vi "niScope Digitizing Process.vi"(8 "error in":errorcluster, 11 "niScope session":variant) -> (0 "error out":errorcluster, 3 "auxiliary data out":variant)   [LabVIEW 2018, in "niScope Virtual Digitizer.lvlib"]
doc: "This is called assynchronously! It is process where niScope digitizers digitize samples, then fetching them and returning them via queue to the calling process. It handles both single shot and continuous sampling. For single shot sampling it returns the data in blocks of predifined size after all sampling is done. For streaming mode it streams the data blocks continuously. In any case the calling process must take the data from queue in parallel with this VI otherwise it will overflow! The function also returnes status in the data packet which may be used to determine progess of the digitizing and state of the memory buffer.\nThis VI also returns auxiliary data, i.e. structure with scaling factors, time stamps and measured temperature during sampling."
uses:
  niScope Virtual Digitizer.lvlib
  niScope Session.ctl
  niScope Virtual Channel Config.ctl
  niScope Virtual Channel Mode.ctl
  niScope Virtual Channel Input Z.ctl
  niScope Virtual Channel Coupling.ctl
  niScope Type.ctl
  niScope Digitizing Process Options.ctl
  niScope Data Packet.ctl
  niScope Trigger Setup.ctl
  <instrlib>/niScope/Controls/niScope trigger coupling.ctl
  <instrlib>/niScope/Controls/niScope trigger slope.ctl
  niScope Record Aux Data.ctl
  <vilib>/Analysis/baseanly.llb/Mean (DBL).vi
  <vilib>/Utility/error.llb/Error Cluster From Error Code.vi
  <instrlib>/niScope/Acquire/Fetch/niScope Fetch Binary 32.vi
  <instrlib>/niScope/Acquire/Fetch/niScope Fetch Binary 16.vi
  <vilib>/ErrorRing/Error Ring.xnode
  <vilib>/Analysis/NI_AALBase.lvlib
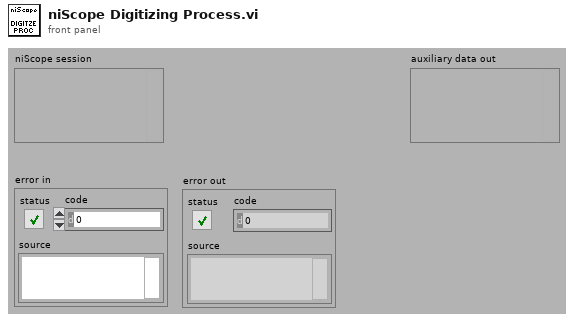
[diagram p1: front panel]
types:
  T1 = typedef "niScope Virtual Digitizer.lvlib/niScope Session.ctl" = cluster{"channel cfg":T2[], "sessions":refnum<k20>[], "multi cards":bool, "channels":i32, "type":T6, "memory [B/chn]":i32, "ext. clock [Hz]":dbl, "samples count":i64, "use streaming":bool, "proc setup":T7, "sample width [B]":i32, "ranges [V]":dbl[], "trigger setup":T8, "fs [Hz]":dbl, "bitres [bit]":i32}
  T2 = typedef "niScope Virtual Digitizer.lvlib/niScope Virtual Channel Config.ctl" = cluster{"Address":refnum<k15>, "Channel":i32, "Mode":T3, "Input Z":T4, "Coupling":T5, "Range [Vpk]":dbl, "btn clr":bool, "btn up":bool, "btn down":bool}
  T3 = typedef "niScope Virtual Digitizer.lvlib/niScope Virtual Channel Mode.ctl" = enum16{"Single ended", "Unbal. differential", "Differential"}
  T4 = typedef "niScope Virtual Digitizer.lvlib/niScope Virtual Channel Input Z.ctl" = enum16{"1 MOhm", "50 Ohm"}
  T5 = typedef "niScope Virtual Digitizer.lvlib/niScope Virtual Channel Coupling.ctl" = enum16{"AC", "DC", "GND"}
  T6 = typedef "niScope Virtual Digitizer.lvlib/niScope Type.ctl" = enum16{"n/a", "5922"}
  T7 = typedef "niScope Virtual Digitizer.lvlib/niScope Digitizing Process Options.ctl" = cluster{"packet size [smpl]":i64, "current timeout [s]":dbl, "blk2blk timeout [s]":dbl, "event time":timestamp, "temp sampl T [s]":dbl, "data queue":refnum<queue>, "stop notifier":refnum<notifier>, "proc ref":refnum<vi>}
  T8 = typedef "niScope Virtual Digitizer.lvlib/niScope Trigger Setup.ctl" = cluster{"coupling":T9, "level [V]":dbl, "slope":T10, "mode":enum16{"Immediate", "External", "Level"}}
  T9 = typedef "niScope trigger coupling.ctl" = u16
  T10 = typedef "niScope trigger slope.ctl" = i32
  T11 = typedef "niScope Virtual Digitizer.lvlib/niScope Data Packet.ctl" = cluster{"int32":i32[][], "card buffer [%]":dbl, "all done?":bool, "offset [smpl]":i64, "sampling?":bool, "queue buffer [%]":dbl, "int16":i16[][], "is int16?":bool, "count [smpl]":i32, "valid?":bool}
  T12 = typedef "niScope Virtual Digitizer.lvlib/niScope Record Aux Data.ctl" = cluster{"T smpl":i64[], "T [deg C]":dbl[][], "time stamp [s]":dbl[], "offset":dbl[], "gain":dbl[], "increment [s]":dbl, "valid?":bool, "abs timestamp":timestamp}
  T13 = cluster{"actualSamples":i32, "absoluteInitialX":dbl, "relativeInitialX":dbl, "xIncrement":dbl, "offset":dbl, "gain":dbl, "reserved1":dbl, "reserved2":dbl}
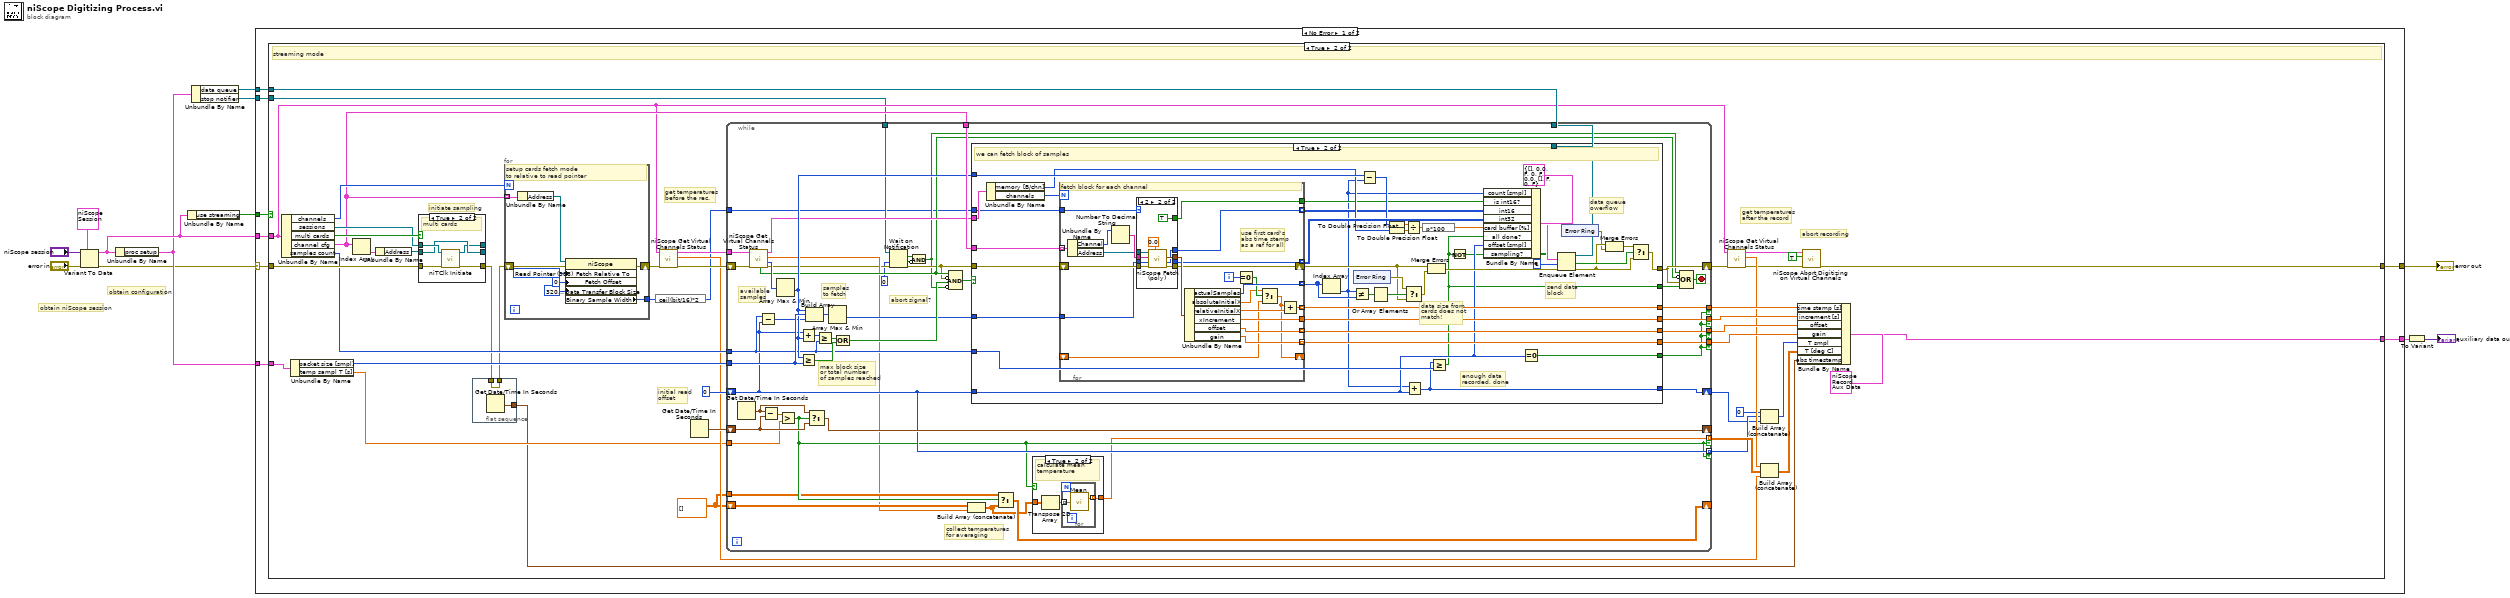
[diagram p0: block diagram]
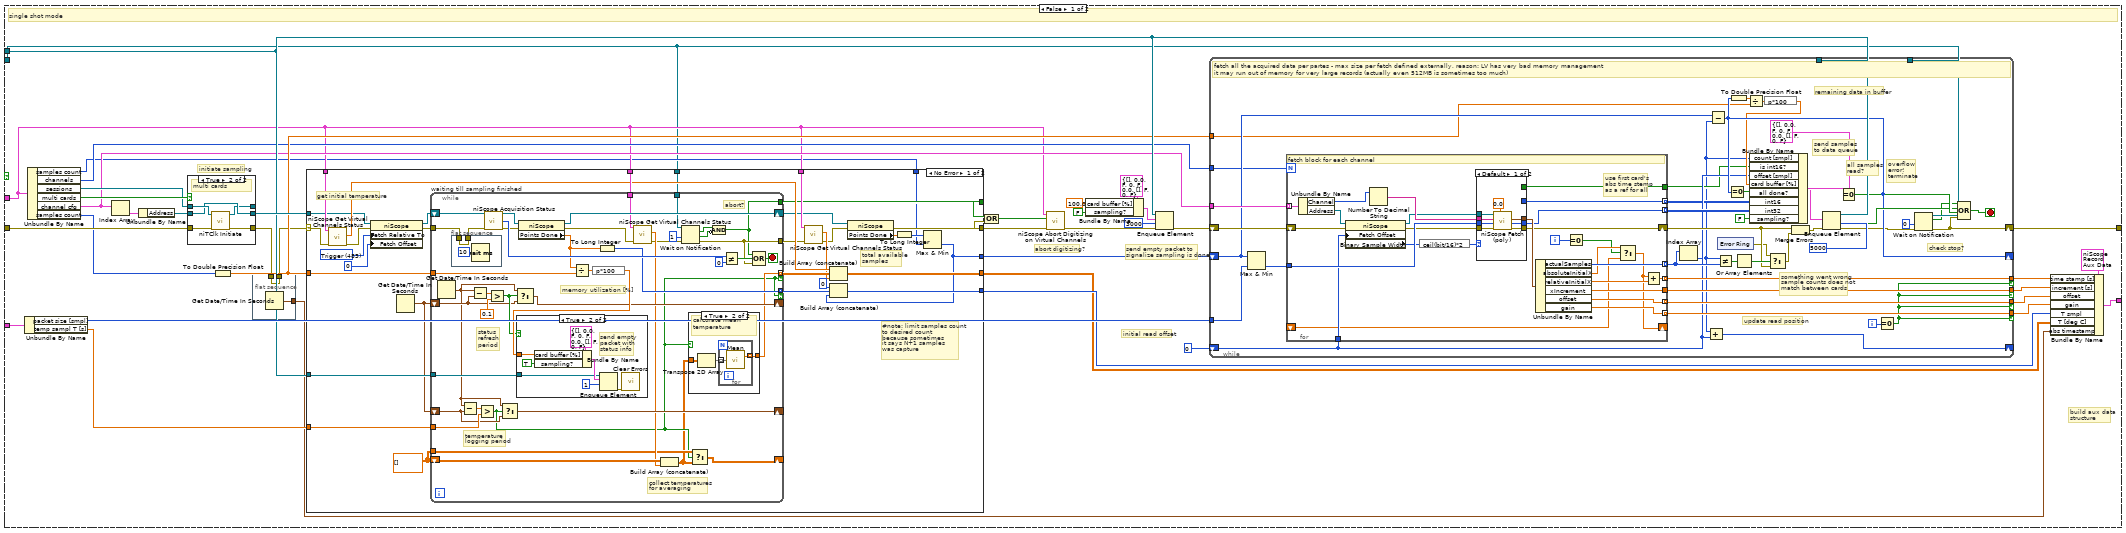
[diagram p2: hidden frame]
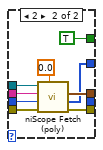
[diagram p3: hidden frame]
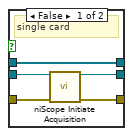
[diagram p7: hidden frame]
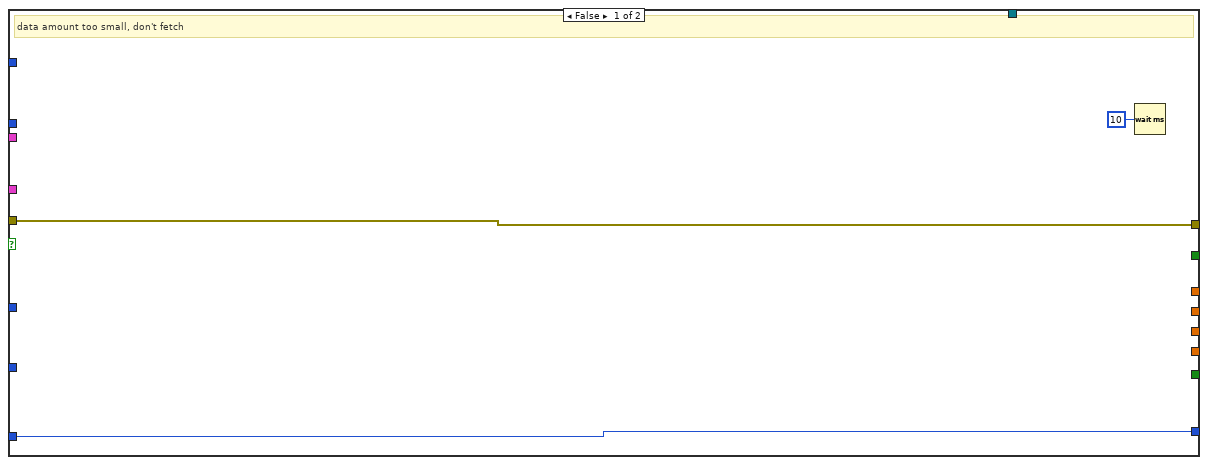
[diagram p9: hidden frame]
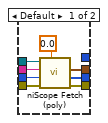
[diagram p10: hidden frame]
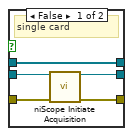
[diagram p11: hidden frame]
diagram:
  # "obtain configuration"
  # "obtain niScope session"
  n1 = Variant To Data(error in="error in", type=T1 {"channel cfg"=[], "sessions"=[], "multi cards"=FALSE, "channels"=0, "type"=enum."n/a", "memory [B/chn]"=0, "ext. clock [Hz]"=0.0, "samples count"=0, "use streaming"=FALSE, "proc setup"={"packet size [smpl]"=0, "current timeout [s]"=0.0, "blk2blk timeout [s]"=0.0, "event time"=timestamp(0 s since 1904-01-01), "temp sampl T [s]"=0.0, "data queue"=refnum, "stop notifier"=refnum, "proc ref"=refnum}, "sample width [B]"=0, "ranges [V]"=[], "trigger setup"={"coupling"=0, "level [V]"=0.0, "slope"=0, "mode"=enum."Immediate"}, "fs [Hz]"=0.0, "bitres [bit]"=0} ("niScope out"), Variant="niScope session") -> (data=w3:T1, error out=w1:errorcluster)
  n2 = Unbundle By Name(w3) -> ("proc setup"=w2:T7)
  n3 = Unbundle By Name(w3) -> ("use streaming"=w12:bool)
  n4 = Unbundle By Name(w2) -> ("data queue"=w6:refnum<queue>, "stop notifier"=w4:refnum<notifier>)
  n5 = case shown="No Error" w1 {
    selector: w1 -> [w14 w469]
    tunnel: w12 -> [w20 _]
    tunnel: w2 -> [w19 _]
    tunnel: w6 -> [w18 _]
    tunnel: [w17 w469] -> w5
    tunnel: w3 -> [w16 _]
    tunnel: [w15 _] -> w8
    tunnel: w4 -> [w13 _]
    frame No Error {
      n6 = case shown="True" w20 {
        tunnel: w16 -> [w29 w283]
        tunnel: w14 -> [w61 w297]
        tunnel: w19 -> [w55 w293]
        tunnel: w18 -> [w41 w288]
        tunnel: [w53 w264] -> w17
        tunnel: [w47 w277] -> w15
        tunnel: w13 -> [w24 w262]
        frame False {
          # "abort digitizing?"
          # "initial read offset"
          # "send empty packet to\nsignalize sampling is done"
          # "build aux data\nstructure"
          # "initiate sampling"
          # "single shot mode"
          n7 = Unbundle By Name(w55) -> ("packet size [smpl]"=w54:i64, "temp sampl T [s]"=w32:dbl)
          n8 = Unbundle By Name(w29) -> ("samples count"=w25:i64, "channels"=w35:i32, "sessions"=w57:refnum<k20>[], "multi cards"=w58:bool, "channel cfg"=w30:T2[], "samples count"=w40:i64)
          n9 = Index Array(array=w30) -> (element=w60:T2)  [unwired: 1 in]
          n10 = Unbundle By Name(w60) -> ("Address"=w59:refnum<k15>)
          n11 = case shown="True" w58 {
            tunnel: [w250 w254] -> w23
            tunnel: [w249 w252] -> w56
            tunnel: w61 -> [w248 w255]
            tunnel: w59 -> [w247 w252]
            tunnel: w57 -> [w246 w253]
            tunnel: [w246 w251] -> _
            frame False {
              # "single card"
              n12 = call <instrlib>:"niScope Initiate Acquisition.vi"("instrument handle"=w247, "error in"=w248) -> ("instrument handle out"=w249:refnum<k15>, "error out"=w250:errorcluster)  [unwired: 12 in]
            }
            frame True {
              # "multi cards"
              n13 = call <instrlib>:"niTClk Initiate.vi"("error in (no error)"=w255, "sessions"=w253) -> ("error out"=w254:errorcluster, "sessions out"=w251:refnum<k20>[])  [unwired: 8 in]
            }
          }
          n14 = To Double Precision Float(number=w40) -> (double precision float=w39:dbl)
          n15 = flat-sequence {
            tunnel: w23 -> [w63]
            tunnel: [w63] -> w22
            tunnel: [w62] -> w21
            frame #0 {
              n16 = Get Date/Time In Seconds() -> (seconds since 1Jan1904=w62:timestamp)
            }
          }
          n17 = case shown="No Error" w22 {
            selector: w22 -> [w184 w245]
            tunnel: w56 -> [w162 _]
            tunnel: [w173 w245] -> w27
            tunnel: w41 -> [w188 _]
            tunnel: w39 -> [w187 _]
            tunnel: w29 -> [w185 _]
            tunnel: w29 -> [w183 _]
            tunnel: [w178 _] -> w38
            tunnel: [w177 _] -> w37
            tunnel: w29 -> [w175 _]
            tunnel: [w158 _] -> w33
            tunnel: w32 -> [w169 _]
            tunnel: w24 -> [w167 _]
            tunnel: [w166 _] -> w26
            tunnel: w25 -> [w157 _]
            frame No Error {
              w161 = 483 items=["Start"=482, "Trigger"=483, "Pretrigger"=477, "Now"=481, "Read Pointer"=388] ("Fetch:Fetch Relative To")
              w168 = dbl[][] []
              # "#note: limit samples count\nto desired count\nbecause sometimes\nit says N+1 samples\nwas capture"
              # "total available\nsamples"
              # "get initial temperature"
              n18 = call "niScope Get Virtual Channels Status.vi"("error in"=w184, "niScope in"=w183) -> ("error out"=w164:errorcluster, "temperatures [deg C]"=w181:dbl[])  [unwired: 5 in, 3 out]
              n19 = property class="niScope"(reference=w162, error in=w164, "Fetch Relative To"=w161, "Fetch Offset"=0 ("Fetch:Fetch Offset")) -> (reference out=w163:refnum<k15>, error out=w165:errorcluster)
              n20 = Get Date/Time In Seconds() -> (seconds since 1Jan1904=w186:timestamp)
              n21 = while "waiting till sampling finished" {
                tunnel: w165 -> [w225]
                tunnel: [w192] -> w176
                shift-right: [w221] -> w171
                shift-left: w163 -> [w230]
                shift-right: [w212] -> _
                shift-left: w186 -> [w213]
                tunnel: w188 -> [w218]
                tunnel: w187 -> [w217]
                shift-right: [w207] -> _
                shift-left: w186 -> [w208]
                tunnel: w169 -> [w210]
                tunnel: w185 -> [w205]
                tunnel: [w198] -> w182 mode=indexing if=w197
                tunnel: [w203] -> w180 mode=indexing if=w197
                shift-right: [w199] -> _
                shift-left: w168 -> [w202]
                tunnel: w168 -> [w200]
                tunnel: w167 -> [w194]
                tunnel: [w189] -> w166
                stop <- w227 stop-if-true
                # "abort?"
                # "collect temperatures\nfor averaging"
                # "temperature\nlogging period"
                # "memory utilization [%]"
                # "status\nrefresh\nperiod"
                n22 = Get Date/Time In Seconds() -> (seconds since 1Jan1904=w209:timestamp)
                n23 = flat-sequence {
                  tunnel: w225 -> [w243]
                  tunnel: [w243] -> w224
                  frame #0 {
                    n24 = Wait (ms)(milliseconds to wait=u32 10) -> ()  [unwired: 1 out]
                  }
                }
                n25 = Subtract(x=w209, y=w208) -> (x-y=w211:dbl)
                n26 = Subtract(x=w209, y=w213) -> (x-y=w220:dbl)
                n27 = Greater?(x=w211, y=w210) -> (0:w197:bool)
                n28 = call <instrlib>:"niScope Acquisition Status.vi"("instrument handle"=w230, "error in"=w224) -> ("instrument handle out"=w222:refnum<k15>, "acquisition status"=w228:i32, "error out"=w223:errorcluster)  [unwired: 11 in]
                n29 = Greater?(x=w220, y=0.1) -> (0:w214:bool)
                n30 = Select(t=w209, s=w197, f=w208) -> (s? t:f=w207:timestamp)
                n31 = Select(t=w209, s=w214, f=w213) -> (s? t:f=w212:timestamp)
                n32 = property class="niScope"(reference=w222, error in=w223) -> (reference out=w221:refnum<k15>, error out=w206:errorcluster, "Points Done"=w204:dbl)
                n33 = Divide(x=w204, y=w217) -> (x/y=w216:dbl)
                n34 = expression code="p*100"(w216) -> (w215:dbl)
                n35 = case shown="True" w214 {
                  tunnel: w218 -> [_ w239]
                  tunnel: w215 -> [_ w237]
                  frame False {
                  }
                  frame True {
                    # "send empty\npacket with\nstatus info"
                    n36 = Bundle By Name(cluster=T11 {"int32"=[], "card buffer [%]"=0.0, "all done?"=FALSE, "offset [smpl]"=0, "sampling?"=FALSE, "queue buffer [%]"=0.0, "int16"=[], "is int16?"=FALSE, "count [smpl]"=0, "valid?"=FALSE} ("element"), "card buffer [%]"=w237, "sampling?"=TRUE) -> (w242:T11)
                    n37 = Enqueue Element(queue=w239, element=w242, timeout in ms (-1)=1) -> (error out=w238:errorcluster)  [unwired: 1 in, 2 out]
                    n38 = call <vilib>:"Clear Errors.vi"("error in (no error)"=w238) -> ()  [unwired: 5 in, 2 out]
                  }
                }
                n39 = To Long Integer(number=w204) -> (32bit integer=w203:i32)
                n40 = call "niScope Get Virtual Channels Status.vi"("error in"=w206, "niScope in"=w205) -> ("error out"=w195:errorcluster, "temperatures [deg C]"=w201:dbl[])  [unwired: 5 in, 3 out]
                n41 = Build Array (concatenate)(w202, w201) -> (w196:dbl[][])
                n42 = Wait on Notification(notifier=w194, timeout in ms (-1)=1, error in (no error)=w195) -> (notification=w191:bool, timed out?=w190:bool, error out=w192:errorcluster)  [unwired: 1 in, 1 out]
                n43 = case shown="True" w197 {
                  tunnel: w196 -> [_ w233]
                  tunnel: [_ w231] -> w198
                  frame False {
                  }
                  frame True {
                    # "calculate mean\ntemperature"
                    n44 = Transpose 2D Array(2D array=w233) -> (transposed array=w232:dbl[][])
                    n45 = for {
                      tunnel: w232 -> [w235] mode=indexing
                      tunnel: [w234] -> w231 mode=indexing
                      n46 = call-poly <vilib>:"Mean.vi"("X"=w235) -> ("mean"=w234:dbl)  [unwired: 1 out]
                    }
                  }
                }
                n47 = Select(t=w200, s=w197, f=w196) -> (s? t:f=w199:dbl[][])
                n48 = Compound Arithmetic op=AND(w191, invert w190) -> (w189:bool)
                n49 = Not Equal?(x=w228, y=i64 0) -> (x != y?=w226:bool)
                n50 = Compound Arithmetic op=OR(w189, w226, w192) -> (w227:bool)
              }
              n51 = call "niScope Get Virtual Channels Status.vi"("error in"=w176, "niScope in"=w175) -> ("error out"=w172:errorcluster, "temperatures [deg C]"=w174:dbl[])  [unwired: 5 in, 3 out]
              n52 = Build Array (concatenate)(w181, w182, w174) -> (w177:dbl[][])
              n53 = property class="niScope"(reference=w171, error in=w172) -> (error out=w173:errorcluster, "Points Done"=w170:dbl)  [unwired: 1 out]
              n54 = To Long Integer(number=w170) -> (32bit integer=w159:i32)
              n55 = Max & Min(x=w159, y=w157) -> (min(x,y)=w158:i64)  [unwired: 1 out]
              n56 = Build Array (concatenate)(0, w180, w158) -> (w178:i64[])
            }
            frame Error {
            }
          }
          n57 = Compound Arithmetic op=OR(w26, w27) -> (w28:bool)
          n58 = call "niScope Abort Digitizing on Virtual Channels.vi"("error in"=w27, "abort (True)"=w28, "niScope in"=w29) -> ("error out"=w31:errorcluster)  [unwired: 7 in, 1 out]
          n59 = Bundle By Name(cluster=T11 {"int32"=[], "card buffer [%]"=0.0, "all done?"=FALSE, "offset [smpl]"=0, "sampling?"=FALSE, "queue buffer [%]"=0.0, "int16"=[], "is int16?"=FALSE, "count [smpl]"=0, "valid?"=FALSE} ("element"), "card buffer [%]"=100.0 ("progress [%]"), "sampling?"=FALSE) -> (w42:T11)
          n60 = Enqueue Element(queue=w41, element=w42, timeout in ms (-1)=3000, error in (no error)=w31) -> (error out=w34:errorcluster)  [unwired: 2 out]
          n61 = while {
            tunnel: w30 -> [w107]
            shift-right: [w80] -> _
            shift-left: w33 -> [w98]
            tunnel: w54 -> [w105]
            tunnel: [w104] -> w50 if=w99
            tunnel: [w103] -> w51 if=w99
            tunnel: [w101] -> w49 if=w99
            tunnel: [w100] -> w48 if=w99
            tunnel: w41 -> [w90]
            shift-right: [w68] -> w53
            shift-left: w34 -> [w106]
            shift-right: [w81] -> _
            shift-left: 0 -> [w72]
            tunnel: w39 -> [w78]
            tunnel: w35 -> [w73]
            tunnel: w24 -> [w66]
            i -> [w102]
            stop <- w85 stop-if-true
            # "check stop?"
            # "remaining data in buffer"
            # "update read position"
            # "overflow\nerror!\nterminate"
            # "send samples\nto data queue"
            # "all samples\nread?"
            # "something went wrong\nsample counts does not\nmatch between cards"
            # "fetch all the acquired data per partes - max size per fetch defined externally, reason: LV has very bad memory management\nit may run out of memory for very large records (actually even 512MB is sometimes too much)"
            n62 = Max & Min(x=w98, y=w105) -> (min(x,y)=w75:i64)  [unwired: 1 out]
            n63 = for {
              N: w73 -> [_]
              tunnel: w107 -> [w139] mode=indexing
              tunnel: w75 -> [w136]
              tunnel: [w134] -> w97 mode=indexing
              tunnel: [w133] -> w82 mode=indexing
              shift-right: [w132] -> w94
              shift-left: w106 -> [w126]
              tunnel: [w130] -> w103 mode=indexing
              tunnel: [w129] -> w104
              tunnel: [w128] -> w101 mode=indexing
              tunnel: [w127] -> w100 mode=indexing
              tunnel: w72 -> [w122]
              tunnel: [w119] -> w71 mode=indexing
              tunnel: [w118] -> w70
              shift-right: [w114] -> _
              shift-left: _ -> [w113]
              i -> [w116]
              # "use first card's\nabs time stemp\nas a ref for all"
              # "fetch block for each channel"
              n64 = Unbundle By Name(w139) -> ("Channel"=w138:i32, "Address"=w124:refnum<k15>)
              n65 = property class="niScope"(reference=w124, error in=w126, "Fetch Offset"=w122) -> (reference out=w123:refnum<k15>, error out=w125:errorcluster, "Binary Sample Width"=w121:i32)
              n66 = Number To Decimal String(number=w138) -> (decimal integer string=w137:string)  [unwired: 1 in]
              n67 = expression code="ceil(bit/16)*2"(w121) -> (w120:i32)
              n68 = case shown="Default" w120 {
                tunnel: w137 -> [w147 w156]
                tunnel: w136 -> [w146 w155]
                tunnel: [w144 w153] -> w135
                tunnel: [w143 _] -> w133
                tunnel: [w142 w152] -> w132
                tunnel: w125 -> [w141 w151]
                tunnel: w123 -> [w140 w150]
                tunnel: [_ w149] -> w119
                tunnel: [_ TRUE] -> w118
                frame Default {
                  n69 = call-poly <instrlib>:"niScope Fetch (poly).vi"("timeout"=0.0, "error in"=w141, "numSamples"=w146, "channels"=w147, "instrument handle"=w140) -> ("error out"=w142:errorcluster, "wfm"=w143:i32[], "wfm info"=w144:T13)  [unwired: 3 in, 1 out]
                }
                frame 2 {
                  n70 = call-poly <instrlib>:"niScope Fetch (poly).vi"("timeout"=0.0, "error in"=w151, "numSamples"=w155, "channels"=w156, "instrument handle"=w150) -> ("error out"=w152:errorcluster, "wfm"=w149:i16[], "wfm info"=w153:T13)  [unwired: 3 in, 1 out]
                }
              }
              n71 = Unbundle By Name(w135) -> ("actualSamples"=w134:i32, "absoluteInitialX"=w117:dbl, "relativeInitialX"=w131:dbl, "xIncrement"=w129:dbl, "offset"=w128:dbl, "gain"=w127:dbl)
              n72 = Equal To 0?(x=w116) -> (x = 0?=w115:bool)
              n73 = Select(t=w117, s=w115, f=w113) -> (s? t:f=w114:dbl)
              n74 = Add(x=w114, y=w131) -> (x+y=w130:dbl)
            }
            n75 = Index Array(array=w97) -> (element=w69:i32)  [unwired: 1 in]
            n76 = Add(x=w69, y=w72) -> (x+y=w81:i32)
            n77 = Subtract(x=w98, y=w69) -> (x-y=w80:i64)
            n78 = Not Equal?(x=w69, y=w97) -> (x != y?=w96:bool[])
            n79 = xnode "Error Ring"() -> ("error out"=w93:errorcluster)
            n80 = Equal To 0?(x=w80) -> (x = 0?=w83:bool)
            n81 = To Double Precision Float(number=w80) -> (double precision float=w79:dbl)
            n82 = Or Array Elements(Boolean array=w96) -> (logical OR=w95:bool)
            n83 = Divide(x=w79, y=w78) -> (x/y=w77:dbl)
            n84 = expression code="p*100"(w77) -> (w76:dbl)
            n85 = Bundle By Name(cluster=T11 {"int32"=[], "card buffer [%]"=0.0, "all done?"=FALSE, "offset [smpl]"=0, "sampling?"=FALSE, "queue buffer [%]"=0.0, "int16"=[], "is int16?"=FALSE, "count [smpl]"=0, "valid?"=FALSE} ("niScope packet"), "count [smpl]"=w69, "is int16?"=w70, "offset [smpl]"=w72, "card buffer [%]"=w76, "all done?"=w83, "int16"=w71, "int32"=w82, "sampling?"=FALSE) -> (w88:T11)
            n86 = Select(t=w93, s=w95, f=w94) -> (s? t:f=w92:errorcluster)
            n87 = Merge Errors(w94, w92) -> (w91:errorcluster)
            n88 = Enqueue Element(queue=w90, element=w88, timeout in ms (-1)=5000, error in (no error)=w91) -> (timed out?=w84:bool, error out=w67:errorcluster)  [unwired: 1 out]
            n89 = Equal To 0?(x=w80) -> (x = 0?=w86:bool)
            n90 = Equal To 0?(x=w102) -> (x = 0?=w99:bool)
            n91 = Wait on Notification(notifier=w66, timeout in ms (-1)=0, error in (no error)=w67) -> (notification=w64:bool, error out=w68:errorcluster)  [unwired: 1 in, 2 out]
            n92 = Compound Arithmetic op=OR(w64, w84, w86, w68) -> (w85:bool)
          }
          n93 = Bundle By Name(cluster=T12 {"T smpl"=[], "T [deg C]"=[], "time stamp [s]"=[], "offset"=[], "gain"=[], "increment [s]"=0.0, "valid?"=FALSE, "abs timestamp"=timestamp(0 s since 1904-01-01)} ("aux data"), "time stamp [s]"=w51, "increment [s]"=w50, "offset"=w49, "gain"=w48, "T smpl"=w38, "T [deg C]"=w37, "abs timestamp"=w21) -> (w47:T12)
        }
        frame True {
          w266 = dbl[][] []
          # "initial read\noffset"
          # "get temperatures\nbefore the rec."
          # "abort recording"
          # "get temperatures\nafter the record"
          # "initiate sampling"
          # "streaming mode"
          n94 = Unbundle By Name(w283) -> ("channels"=w294:i32, "sessions"=w295:refnum<k20>[], "multi cards"=w296:bool, "channel cfg"=w289:T2[], "samples count"=w290:i64)
          n95 = Unbundle By Name(w293) -> ("packet size [smpl]"=w292:i64, "temp sampl T [s]"=w267:dbl)
          n96 = Index Array(array=w289) -> (element=w299:T2)  [unwired: 1 in]
          n97 = Unbundle By Name(w299) -> ("Address"=w298:refnum<k15>)
          n98 = case shown="True" w296 {
            tunnel: [w463 w467] -> w259
            tunnel: [w462 w465] -> _
            tunnel: w297 -> [w461 w468]
            tunnel: w298 -> [w460 w465]
            tunnel: w295 -> [w459 w466]
            tunnel: [w459 w464] -> _
            frame False {
              # "single card"
              n99 = call <instrlib>:"niScope Initiate Acquisition.vi"("instrument handle"=w460, "error in"=w461) -> ("instrument handle out"=w462:refnum<k15>, "error out"=w463:errorcluster)  [unwired: 12 in]
            }
            frame True {
              # "multi cards"
              n100 = call <instrlib>:"niTClk Initiate.vi"("error in (no error)"=w468, "sessions"=w466) -> ("error out"=w467:errorcluster, "sessions out"=w464:refnum<k20>[])  [unwired: 8 in]
            }
          }
          n101 = flat-sequence {
            tunnel: w259 -> [w301]
            tunnel: [w301] -> w258
            tunnel: [w300] -> w257
            frame #0 {
              n102 = Get Date/Time In Seconds() -> (seconds since 1Jan1904=w300:timestamp)
            }
          }
          n103 = for {
            N: w294 -> [_]
            shift-right: [w455] -> w287
            shift-left: w258 -> [w458]
            tunnel: w289 -> [w454] mode=indexing
            tunnel: [w451] -> w261
            w457 = 388 items=["Start"=482, "Trigger"=483, "Pretrigger"=477, "Now"=481, "Read Pointer"=388] ("Fetch:Fetch Relative To")
            # "setup cards fetch mode\nto relative to read pointer"
            n104 = Unbundle By Name(w454) -> ("Address"=w453:refnum<k15>)
            n105 = property class="niScope"(reference=w453, error in=w458, "Fetch Relative To"=w457, "Fetch Offset"=0 ("Fetch:Fetch Offset"), "Data Transfer Block Size"=32000000 ("Fetch:Data Transfer Block Size")) -> (error out=w455:errorcluster, "Binary Sample Width"=w451:i32)  [unwired: 1 out]
          }
          n106 = expression code="ceil(bit/16)*2"(w261) -> (w260:i32)
          n107 = call "niScope Get Virtual Channels Status.vi"("error in"=w287, "niScope in"=w283) -> ("error out"=w286:errorcluster, "temperatures [deg C]"=w273:dbl[], "niScope out"=w285:T1)  [unwired: 5 in, 2 out]
          n108 = Get Date/Time In Seconds() -> (seconds since 1Jan1904=w276:timestamp)
          n109 = while {
            shift-right: [w326] -> w284
            shift-left: w286 -> [w349]
            tunnel: w292 -> [w342]
            shift-right: [w334] -> w270
            shift-left: i64 0 -> [w320]
            tunnel: w290 -> [w337]
            tunnel: w289 -> [w343]
            tunnel: w288 -> [w339]
            tunnel: w285 -> [w336]
            tunnel: [w333] -> w281 if=w328
            tunnel: [w332] -> w280 if=w328
            tunnel: [w331] -> w279 if=w328
            tunnel: [w330] -> w278 if=w328
            shift-right: [w321] -> _
            shift-left: w276 -> [w322]
            tunnel: [w314] -> w275 mode=indexing if=w317
            tunnel: [w320] -> w272 mode=indexing if=w317
            tunnel: w267 -> [w318]
            shift-right: [w315] -> _
            shift-left: w266 -> [w313]
            tunnel: w266 -> [w316]
            tunnel: w262 -> [w309]
            tunnel: w260 -> [w302]
            stop <- w329 stop-if-true
            # "abort signal?"
            # "collect temperatures\nfor averaging"
            # "samples\nto fetch"
            # "max block size\nor total number\nof samples reached"
            # "available\nsamples"
            n110 = Get Date/Time In Seconds() -> (seconds since 1Jan1904=w323:timestamp)
            n111 = call "niScope Get Virtual Channels Status.vi"("error in"=w349, "niScope in"=w336) -> ("error out"=w310:errorcluster, "points done"=w348:i64[], "temperatures [deg C]"=w312:dbl[], "niScope out"=w335:T1, "all channels sampling?"=w325:bool)  [unwired: 5 in]
            n112 = Subtract(x=w337, y=w320) -> (x-y=w319:i64)
            n113 = Subtract(x=w323, y=w322) -> (x-y=w324:dbl)
            n114 = Array Max & Min(array=w348) -> (min value=w338:i64)  [unwired: 3 out]
            n115 = Greater?(x=w324, y=w318) -> (0:w317:bool)
            n116 = Add(x=w320, y=w338) -> (x+y=w347:i64)
            n117 = Greater Or Equal?(x=w338, y=w342) -> (x >= y?=w345:bool)
            n118 = Build Array(w338, w342, w319) -> (w341:i64[])
            n119 = Select(t=w323, s=w317, f=w322) -> (s? t:f=w321:timestamp)
            n120 = Greater Or Equal?(x=w347, y=w337) -> (x >= y?=w346:bool)
            n121 = Array Max & Min(array=w341) -> (min value=w340:i64)  [unwired: 3 out]
            n122 = Compound Arithmetic op=OR(w346, w345) -> (w344:bool)
            n123 = Wait on Notification(notifier=w309, timeout in ms (-1)=0, error in (no error)=w310) -> (notification=w306:bool, timed out?=w305:bool, error out=w308:errorcluster)  [unwired: 1 in, 1 out]
            n124 = Compound Arithmetic op=AND(w306, invert w305) -> (w304:bool)
            n125 = Compound Arithmetic op=AND(w325, invert w308, w344, invert w304) -> (w307:bool)
            n126 = Build Array (concatenate)(w313, w312) -> (w311:dbl[][])
            n127 = case shown="True" w307 {
              tunnel: w308 -> [w356 w400]
              tunnel: w343 -> [_ w399]
              tunnel: w340 -> [_ w397]
              tunnel: w339 -> [_ w389]
              tunnel: w338 -> [_ w381]
              tunnel: w337 -> [_ w379]
              tunnel: w320 -> [w357 w370]
              tunnel: w335 -> [_ w376]
              tunnel: [w357 w371] -> w334
              tunnel: [w356 w365] -> w326
              tunnel: [_ w375] -> w333
              tunnel: [_ w374] -> w332
              tunnel: [_ w373] -> w331
              tunnel: [_ w372] -> w330
              tunnel: [_ w369] -> w328
              tunnel: [_ w362] -> w327
              tunnel: w302 -> [_ w361]
              frame False {
                # "data amount too small, don't fetch"
                n128 = Wait (ms)(milliseconds to wait=u32 10) -> ()  [unwired: 1 out]
              }
              frame True {
                # "data queue\nowerflow"
                # "send data\nblock"
                # "data size from\ncards does not\nmatch!"
                # "enough data\nrecorded, done"
                # "we can fetch block of samples"
                n129 = Unbundle By Name(w376) -> ("memory [B/chn]"=w378:i32, "channels"=w398:i32)
                n130 = for {
                  N: w398 -> [_]
                  tunnel: w399 -> [w433] mode=indexing
                  tunnel: [w429] -> w391 mode=indexing
                  tunnel: [w428] -> w386 mode=indexing
                  shift-right: [w427] -> w392
                  shift-left: w400 -> [w421]
                  tunnel: [w425] -> w375 mode=indexing
                  tunnel: [w424] -> w374
                  tunnel: [w423] -> w373 mode=indexing
                  tunnel: [w422] -> w372 mode=indexing
                  tunnel: w397 -> [w419]
                  tunnel: w361 -> [w418]
                  tunnel: [w417] -> w360 mode=indexing
                  tunnel: [w416] -> w359
                  shift-right: [w413] -> _
                  shift-left: _ -> [w412]
                  i -> [w411]
                  # "use first card's\nabs time stemp\nas a ref for all"
                  # "fetch block for each channel"
                  n131 = Unbundle By Name(w433) -> ("Channel"=w432:i32, "Address"=w420:refnum<k15>)
                  n132 = Number To Decimal String(number=w432) -> (decimal integer string=w431:string)  [unwired: 1 in]
                  n133 = case shown="2" w418 {
                    tunnel: w431 -> [w441 w450]
                    tunnel: [w439 w448] -> w430
                    tunnel: [w438 _] -> w428
                    tunnel: [w437 w447] -> w427
                    tunnel: w421 -> [w436 w446]
                    tunnel: w420 -> [w435 w445]
                    tunnel: w419 -> [w434 w444]
                    tunnel: [_ w443] -> w417
                    tunnel: [_ TRUE] -> w416
                    frame Default {
                      n134 = call-poly <instrlib>:"niScope Fetch (poly).vi"("timeout"=0.0, "error in"=w436, "numSamples"=w434, "channels"=w441, "instrument handle"=w435) -> ("error out"=w437:errorcluster, "wfm"=w438:i32[], "wfm info"=w439:T13)  [unwired: 3 in, 1 out]
                    }
                    frame 2 {
                      n135 = call-poly <instrlib>:"niScope Fetch (poly).vi"("timeout"=0.0, "error in"=w446, "numSamples"=w444, "channels"=w450, "instrument handle"=w445) -> ("error out"=w447:errorcluster, "wfm"=w443:i16[], "wfm info"=w448:T13)  [unwired: 3 in, 1 out]
                    }
                  }
                  n136 = Unbundle By Name(w430) -> ("actualSamples"=w429:i32, "absoluteInitialX"=w414:dbl, "relativeInitialX"=w426:dbl, "xIncrement"=w424:dbl, "offset"=w423:dbl, "gain"=w422:dbl)
                  n137 = Equal To 0?(x=w411) -> (x = 0?=w415:bool)
                  n138 = Select(t=w414, s=w415, f=w412) -> (s? t:f=w413:dbl)
                  n139 = Add(x=w413, y=w426) -> (x+y=w425:dbl)
                }
                n140 = Index Array(array=w391) -> (element=w358:i32)  [unwired: 1 in]
                n141 = Not Equal?(x=w358, y=w391) -> (x != y?=w396:bool[])
                n142 = xnode "Error Ring"() -> ("error out"=w394:errorcluster)
                n143 = Subtract(x=w381, y=w358) -> (x-y=w380:i64)
                n144 = Or Array Elements(Boolean array=w396) -> (logical OR=w395:bool)
                n145 = To Double Precision Float(number=w380) -> (double precision float=w385:dbl)
                n146 = To Double Precision Float(number=w378) -> (double precision float=w382:dbl)
                n147 = Divide(x=w385, y=w382) -> (x/y=w384:dbl)
                n148 = Select(t=w394, s=w395, f=w392) -> (s? t:f=w393:errorcluster)
                n149 = Add(x=w358, y=w370) -> (x+y=w371:i64)
                n150 = expression code="p*100"(w384) -> (w383:dbl)
                n151 = Merge Errors(w392, w393) -> (w390:errorcluster)
                n152 = Greater Or Equal?(x=w371, y=w379) -> (x >= y?=w362:bool)
                n153 = Not(x=w362) -> (.not. x?=w363:bool)
                n154 = Bundle By Name(cluster=T11 {"int32"=[], "card buffer [%]"=0.0, "all done?"=FALSE, "offset [smpl]"=0, "sampling?"=FALSE, "queue buffer [%]"=0.0, "int16"=[], "is int16?"=FALSE, "count [smpl]"=0, "valid?"=FALSE} ("niScope packet"), "count [smpl]"=w358, "is int16?"=w359, "int16"=w360, "int32"=w386, "card buffer [%]"=w383, "all done?"=w362, "offset [smpl]"=w370, "sampling?"=w363) -> (w387:T11)
                n155 = Equal To 0?(x=w370) -> (x = 0?=w369:bool)
                n156 = Enqueue Element(queue=w389, element=w387, timeout in ms (-1)=1, error in (no error)=w390) -> (timed out?=w368:bool, error out=w366:errorcluster)  [unwired: 1 out]
                n157 = xnode "Error Ring"() -> ("error out"=w364:errorcluster)
                n158 = Merge Errors(w366, w364) -> (w367:errorcluster)
                n159 = Select(t=w367, s=w368, f=w366) -> (s? t:f=w365:errorcluster)
              }
            }
            n160 = Select(t=w316, s=w317, f=w311) -> (s? t:f=w315:dbl[][])
            n161 = case shown="True" w317 {
              tunnel: w311 -> [_ w352]
              tunnel: [_ w350] -> w314
              frame False {
              }
              frame True {
                # "calculate mean\ntemperature"
                n162 = Transpose 2D Array(2D array=w352) -> (transposed array=w351:dbl[][])
                n163 = for {
                  tunnel: w351 -> [w354] mode=indexing
                  tunnel: [w353] -> w350 mode=indexing
                  n164 = call-poly <vilib>:"Mean.vi"("X"=w354) -> ("mean"=w353:dbl)  [unwired: 1 out]
                }
              }
            }
            n165 = Compound Arithmetic op=OR(w304, invert w325, w326, w327) -> (w329:bool)
          }
          n166 = call "niScope Get Virtual Channels Status.vi"("error in"=w284, "niScope in"=w283) -> ("error out"=w265:errorcluster, "temperatures [deg C]"=w274:dbl[], "niScope out"=w263:T1)  [unwired: 5 in, 2 out]
          n167 = Build Array (concatenate)(i64 0, w272, w270) -> (w269:i64[])
          n168 = Build Array (concatenate)(w274, w275, w273) -> (w268:dbl[][])
          n169 = Bundle By Name(cluster=T12 {"T smpl"=[], "T [deg C]"=[], "time stamp [s]"=[], "offset"=[], "gain"=[], "increment [s]"=0.0, "valid?"=FALSE, "abs timestamp"=timestamp(0 s since 1904-01-01)} ("aux data"), "time stamp [s]"=w281, "increment [s]"=w280, "offset"=w279, "gain"=w278, "T smpl"=w269, "T [deg C]"=w268, "abs timestamp"=w257) -> (w277:T12)
          n170 = call "niScope Abort Digitizing on Virtual Channels.vi"("error in"=w265, "abort (True)"=TRUE, "niScope in"=w263) -> ("error out"=w264:errorcluster)  [unwired: 7 in, 1 out]
        }
      }
    }
    frame Error {
    }
  }
  "error out" <- w5
  n171 = To Variant(anything=w8) -> (Variant=→"auxiliary data out":variant)
